vi "7.4.vi"() -> ()   [LabVIEW 2017]
panel:
  out "强度图":dbl[][](graph)
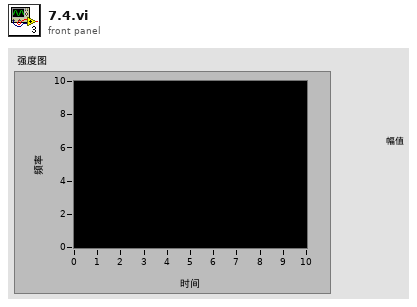
[diagram p1: front panel]
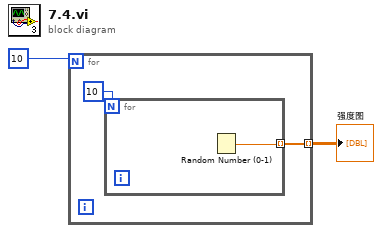
[diagram p0: block diagram]
diagram:
  n1 = for {
    N: 10 -> [_]
    tunnel: [w3] -> w1 mode=indexing
    n2 = for {
      N: 10 -> [_]
      tunnel: [w5] -> w3 mode=indexing
      n3 = Random Number (0-1)() -> (number: 0 to 1=w5:dbl)
    }
  }
  "强度图" <- w1
